vi "4Pi Focus Lock_ids_v1.vi"(7 "Calling VI Ref":refnum<vi>) -> ()   [LabVIEW 2021]
uses:
  4Pi Focus Lock Controls/4Pi Focus Lock - Notifier Type.ctl
  4Pi Focus Lock Controls/4Pi Focus Lock - Actions.ctl
  <vilib>/vision/Image Controls.llb/IMAQ Image.ctl
  <vilib>/Utility/miscctls.llb/LVPointTypeDef.ctl
  Hardware Configuration/Hardware Configuration Controls/Device Type.ctl
  Hardware Configuration/Hardware Configuration Controls/Device Function.ctl
  4Pi Objective Lock - EMBL/4Pi Objective Lock Type Defs/4Pi Obj Lock - Camera Settings.ctl
  Device Library/Cameras/Camera Controls/Generic Camera ROI.ctl
  Device Library/Cameras/Camera Controls/Generic Camera Actions.ctl
  Device Manager/Common Device Queue/Common Device Controls/Common Device Actions.ctl
  Device Library/Stages/Stages Controls/Stage Actions.ctl
  <vilib>/addons/control/pid/pid.llb/PID (DBL).vi
  <vilib>/vision/NI_Vision_Development_Module.lvlib
  <vilib>/addons/control/pid/NI_PID_pid.lvlib
panel:
  in  "Main Tab":enum32{"Acquisition", "Settings", "Gauss fit"}(tab)
  in  "Start Lock":bool
  out "Z Target and Fit Value (µm)":T1(graph)
  out "Stage Position (µm)":dbl=1.0 format="%.2g"
  out "Target Z (µm)":dbl=1.0 format="%.3g"
  out "Measured Z (µm)":dbl=1.0 format="%.3g"
  out "dt (s)":dbl format="%.3f"
  out "dz":dbl format="%.2f"
  out "Z Move":bool
  out "Measured X Position cc (px)":dbl=1.0 format="%.3g"
  out "Measured Y Position cc (px)":dbl=1.0 format="%.3g"
  out "Target Y Position cc (px)":dbl=1.0 format="%.3g"
  out "Target X Position cc (px)":dbl=1.0 format="%.3g"
  out "cc max":dbl=1.0 format="%.3g"
  out "X Y Fit Value (µm)":cluster{dbl, dbl, dbl, dbl, dbl}(graph)
  out "CC Max":cluster{" cc max":dbl}(graph)
  in  "Camera Settings":bool
  in  "Set Camera ROI":bool
  in  "P (Proportional)":dbl=2.0
  in  "I (Integral)":dbl
  in  "D (Derivative)":dbl
  in  "Z Correction Active":bool=TRUE
  in  "Z Move Limit (µm)":dbl=2.0
  in  "Z Drift Threshold (µm)":dbl=2.0
  in  "Sample Z Step Size (µm)":dbl=2.0
  in  "Sample Z Step No.":u32=2
  in  "Update Scale Factor":dbl=2.0
  in  "Frame Accumulation":u32=5
  in  "Pixe Size in XY (µm)":dbl=1.0
  out "Target sx/sy":dbl=1.0 format="%.3g"
  out "Target X Position G (px)":dbl=1.0 format="%.3g"
  out "Target Y Position G (px)":dbl=1.0 format="%.3g"
  out "Measured sx/sy":dbl=1.0 format="%.3g"
  out "Measured X Position G (px)":dbl=1.0 format="%.3g"
  out "Measured Y Position G (px)":dbl=1.0 format="%.3g"
  in  "Metric scale sx/sy":dbl=0.25
  in  "Quit":bool
  # "Z Drift Settings"
  # "PID Control Values"
  # "General Settings"
  # "Conversion to micron"
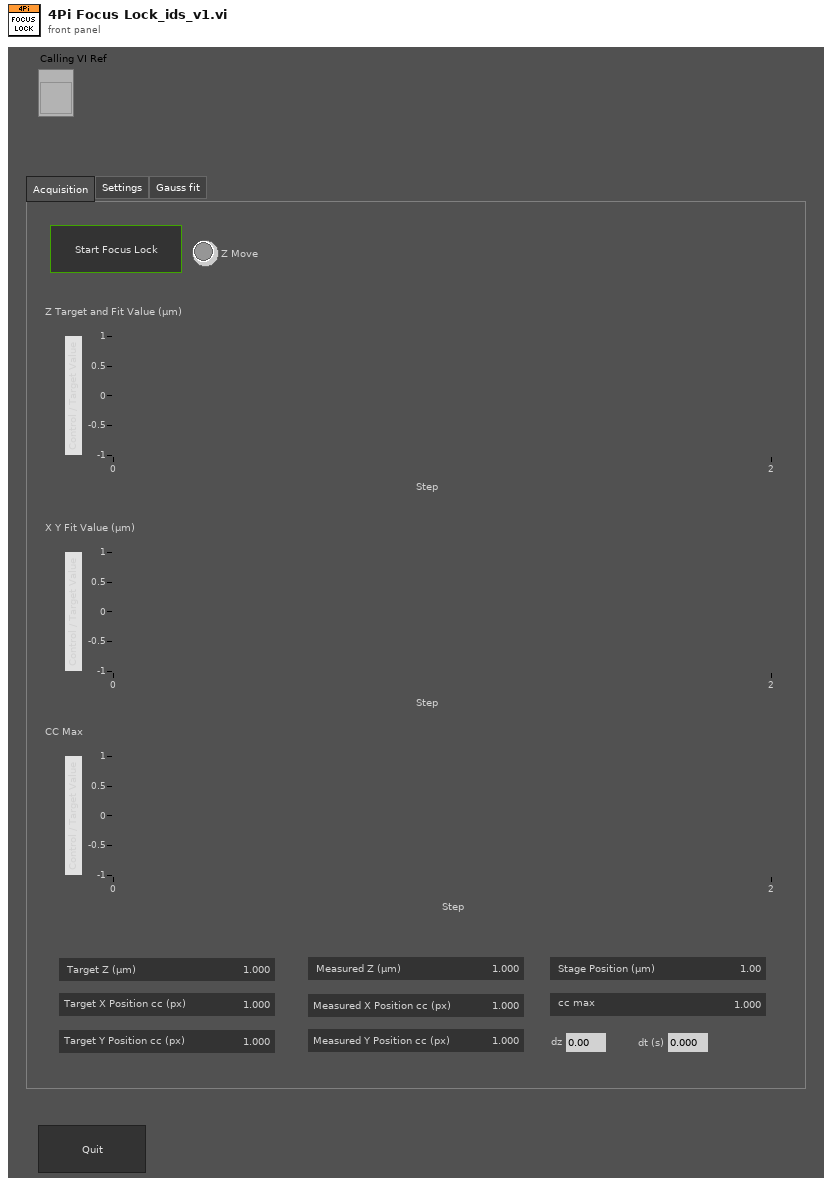
[diagram p1: front panel]
types:
  T1 = cluster{"Target 01":dbl, dbl, dbl, "Current 1":dbl, "Current 2":dbl, "Stage Position":dbl}
  T2 = typedef "4Pi Obj Lock - Camera Settings.ctl" = cluster{"Exposure Time (s)":dbl, "H Offset":u16, "V Offset":u16, "H Width":u16, "V Width":u16}
  T3 = typedef "Device Function.ctl" = enum16{"Primary", "Secondary", "Overview", "Wide Field Drift Correction", "642 nm Excitation", "560 nm Excitation", "940 nm Excitation", "546 nm Excitation", "488 nm Excitation", "405 nm Excitation", "Objective Drift Correction", "4Pi Focus Lock", "4Pi Objective Lock", "Objective XY", "Objective Z", "Sample XY", "Sample Coarse Z", "Sample Z", "4Pi Lower", "4Pi Upper", "Em Small", "Em Large", "Ex Small", "Ex Large", "Mojo", "Adj Cavity", "Line Scanning", "Alert"}
  T4 = typedef "Device Type.ctl" = enum16{"AOTF", "Camera", "Deformable Mirror", "Laser", "Flip Mirror", "Shutter", "Stage", "Waveform", "FPGA", "Email"}
  T5 = enum16{"Always On", "Always Off", "Off While Running"}
  T6 = typedef "LVPointTypeDef.ctl" = cluster{"Horizontal":i16, "Vertical":i16}
  T7 = typedef "4Pi Focus Lock - Actions.ctl" = enum16{"Idle", "Start Lock", "Restart Lock", "Get Target Position", "Get Ref Stack", "Cal Ref FFT", "Get Target Position Gauss", "Move To Init Z", "Start Primary Camera", "Get Current Position Gauss", "Get Current Position", "Get Current XY Position", "Get Current Position 1", "Get Actual Position", "Check Drift Gauss", "Check Drift", "Move Z", "Update Plots", "Delay", "Abort", "Exit Loop", "Quit"}
  T8 = typedef "4Pi Focus Lock - Notifier Type.ctl" = cluster{"Actions":T7, "Z Drift Threshold":dbl, "Z Stage Move Limit (µm)":dbl, "Abort If Error":bool, "Z Correction Active":bool, "PID Values":dbl[], "Running?":bool, "Update Delay (ms)":i32, "Z Step Size (µm)":dbl, "Z Step No.":u32, "No. of Frames":u32, "Ref Stack (SGL)":T9[], "Cur Image (SGL)":T9, "CC Image (SGL) ":T9, "Sample Z (µm)":dbl[], "Initial Z Position (µm)":dbl, "Ref FFT Stack (CSG)":T9[], "Tmp Image FFT (CSG) ":T9[], "CC Image Max (SGL)":T9}
  T9 = typedef "IMAQ Image.ctl" = refnum<image>
  T10 = typedef "Image Type" = u32
  T11 = typedef "Generic Camera Actions.ctl" = enum16{"Status", "Live Preview", "Capture", "Abort", "Set Exposure Time (s)", "Get Exposure Time (s)", "Record Settings", "Set ROI", "Get ROI", "Defect Correction On/Off", "Cooler On/Off", "Fan On/Off", "Quit"}
  T12 = typedef "Generic Camera ROI.ctl" = cluster{"H_Offset":u16, "V_Offset":u16, "H_Width":u16, "V_Width":u16}
  T13 = typedef "Common Device Actions.ctl" = enum16{"Specific Action", "Open Front Panel", "Close Front Panel", "Quit", "Quit All"}
  T14 = cluster{"Target 01":dbl, dbl, dbl, "Current 1":dbl, "Current 2":dbl, "Stage Position":dbl}[]
  T15 = typedef "Stage Actions.ctl" = enum16{"Get Position", "SERVO OFF", "SERVO ON", "SERVO ON/OFF", "MVR", "MOVE", "HALT", "ONTARGET", "ERROR", "REFERENCE", "INIT", "VELOCITY", "STATUS", "EXIT", "HOME", "ZEROPOS", "NANOPOS", "ANALOG", "QUIT"}
  T16 = typedef "Stage Status.ctl" = enum16{"Error", "Abort", "Busy", "On Target"}
  T17 = typedef "2D Gaussian - Best Fit Parameters.ctl" = cluster{"Amplitude":dbl, "X Position":dbl, "Y Position":dbl, "X Width":dbl, "Y Width":dbl, "Offset":dbl}
  T18 = cluster{"PID Values[0]":dbl, "PID Values[1]":dbl, "PID Values[2]":dbl}
  T19 = typedef "LVRectTypeDef.ctl" = cluster{"Left":i16, "Top":i16, "Right":i16, "Bottom":i16}
  T20 = typedef "LVBoundsTypeDef.ctl" = cluster{"Width":u32, "Height":u32}
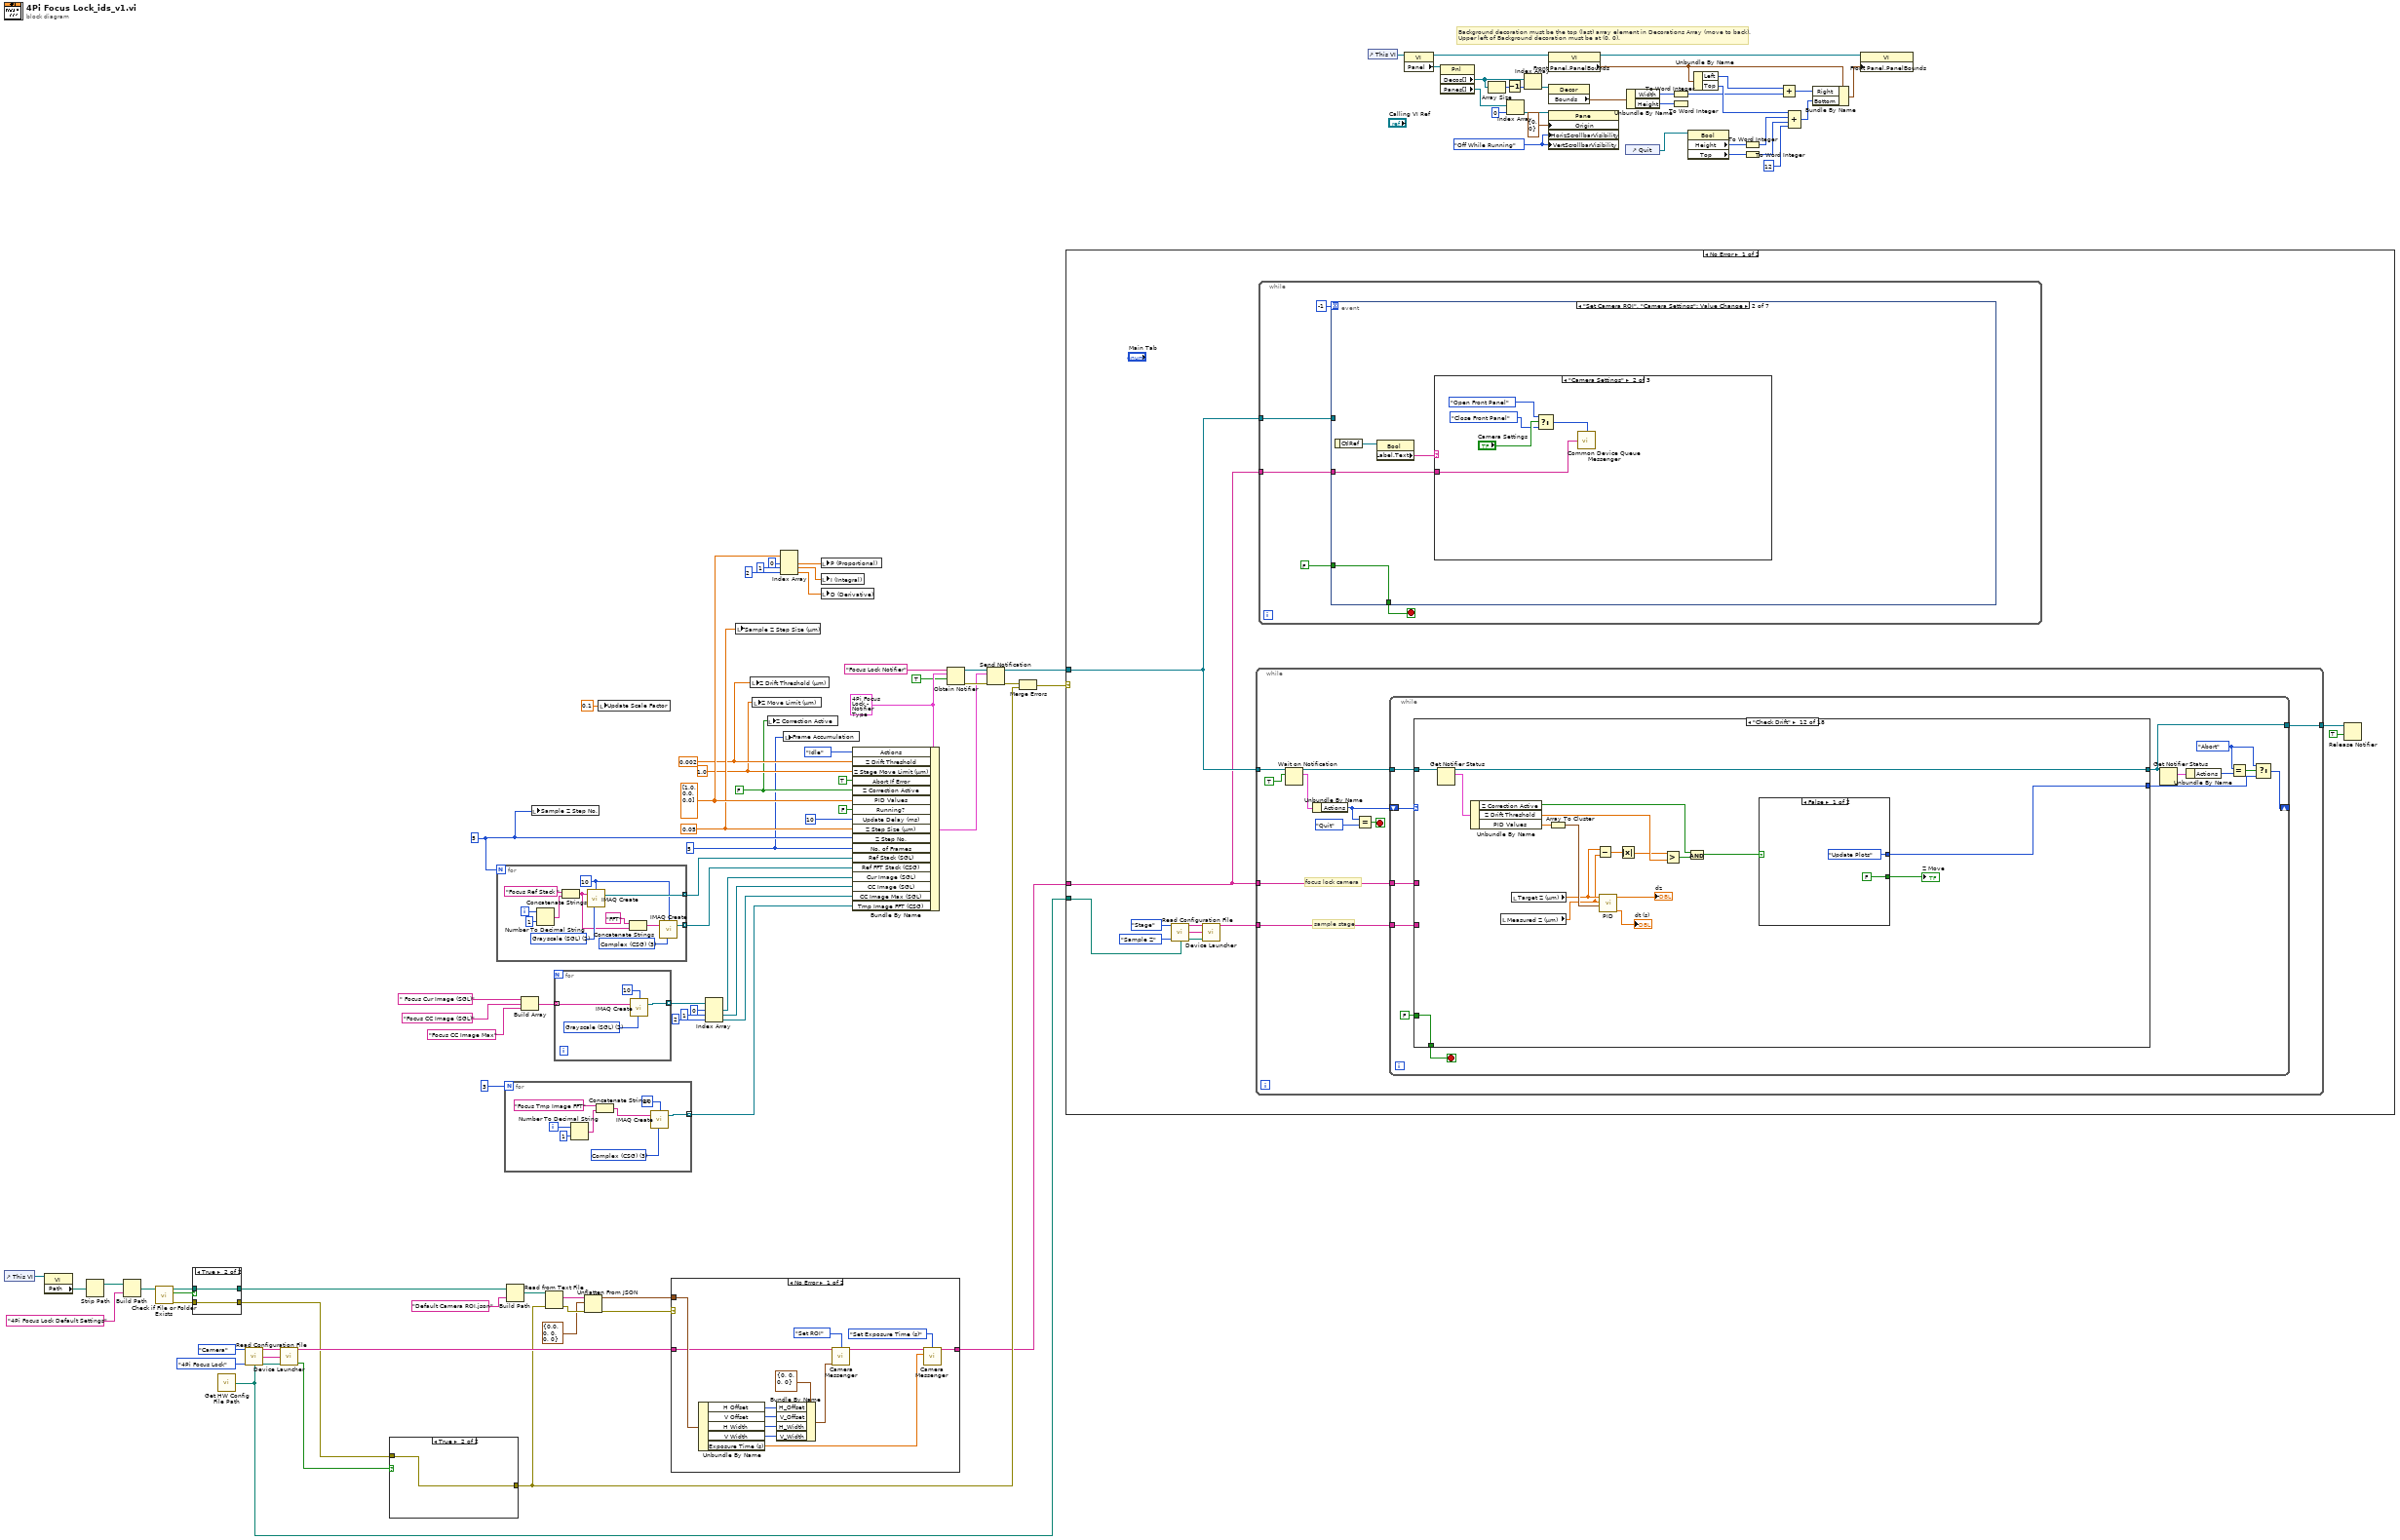
[diagram p0: block diagram]
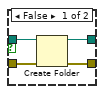
[diagram p2: hidden frame]
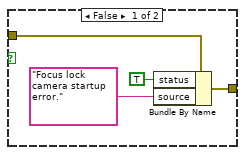
[diagram p3: hidden frame]
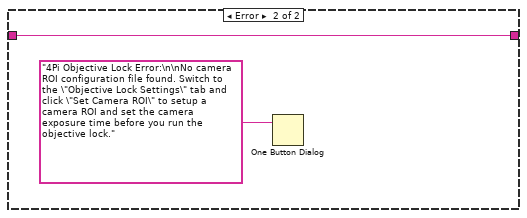
[diagram p4: hidden frame]
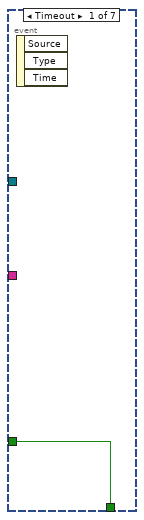
[diagram p5: hidden frame]
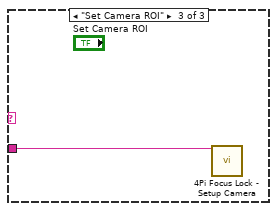
[diagram p7: hidden frame]
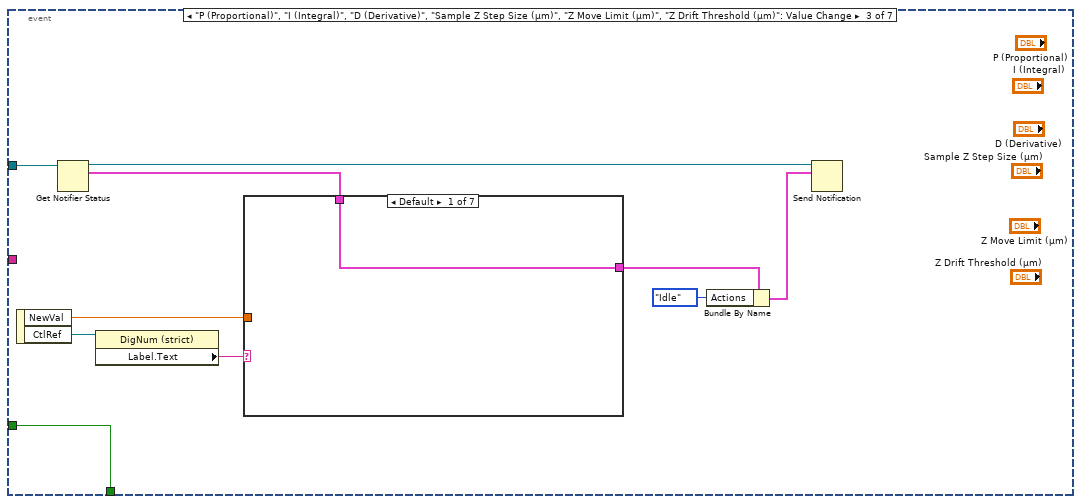
[diagram p8: hidden frame]
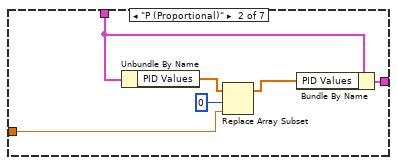
[diagram p9: hidden frame]
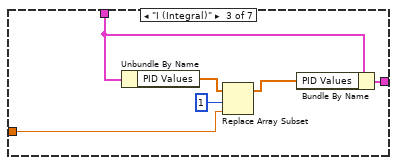
[diagram p10: hidden frame]
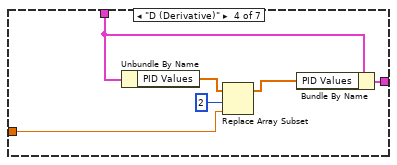
[diagram p11: hidden frame]
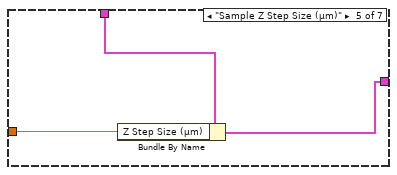
[diagram p12: hidden frame]
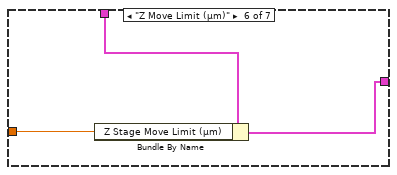
[diagram p13: hidden frame]
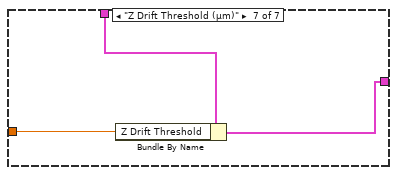
[diagram p14: hidden frame]
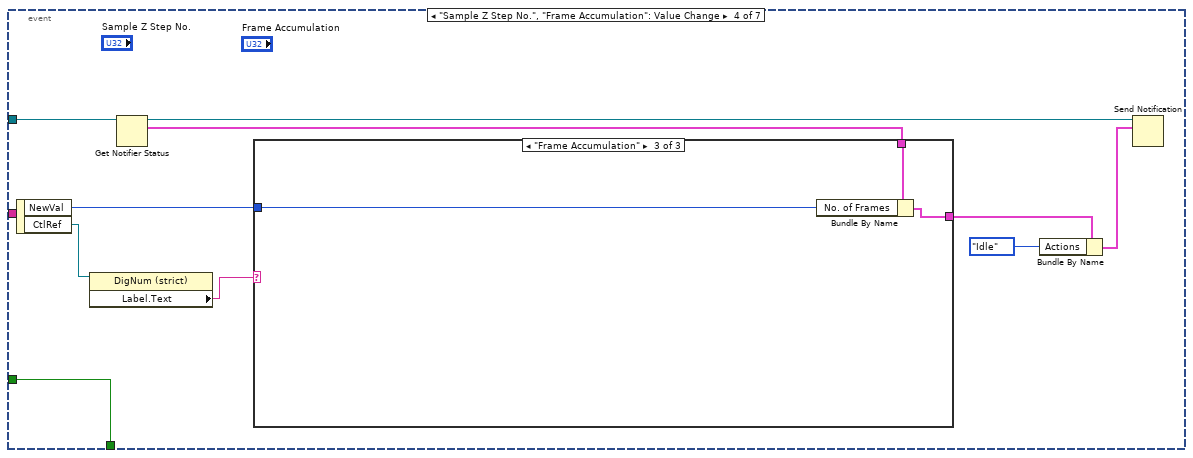
[diagram p15: hidden frame]
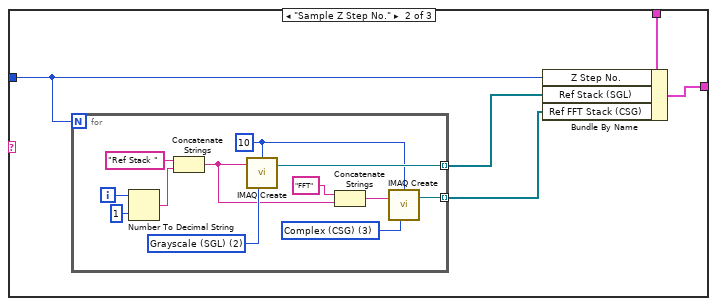
[diagram p17: hidden frame]
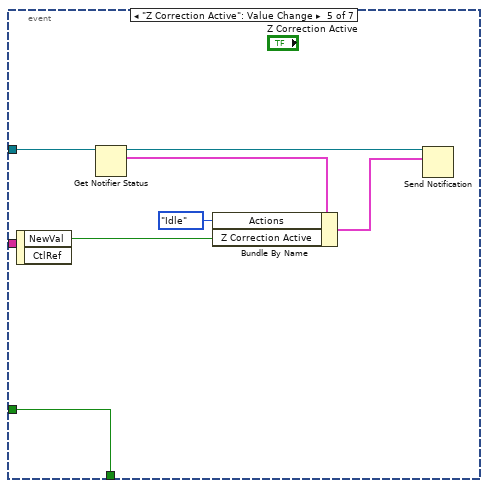
[diagram p18: hidden frame]
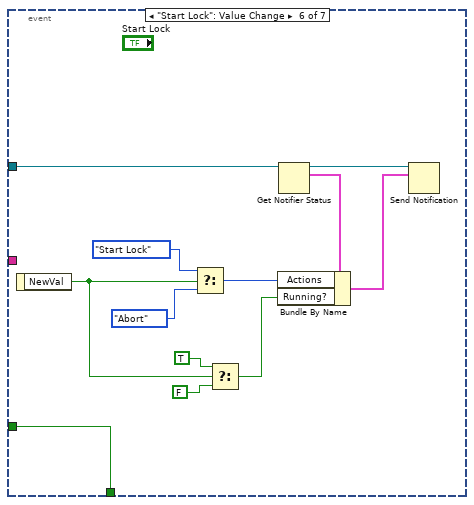
[diagram p19: hidden frame]
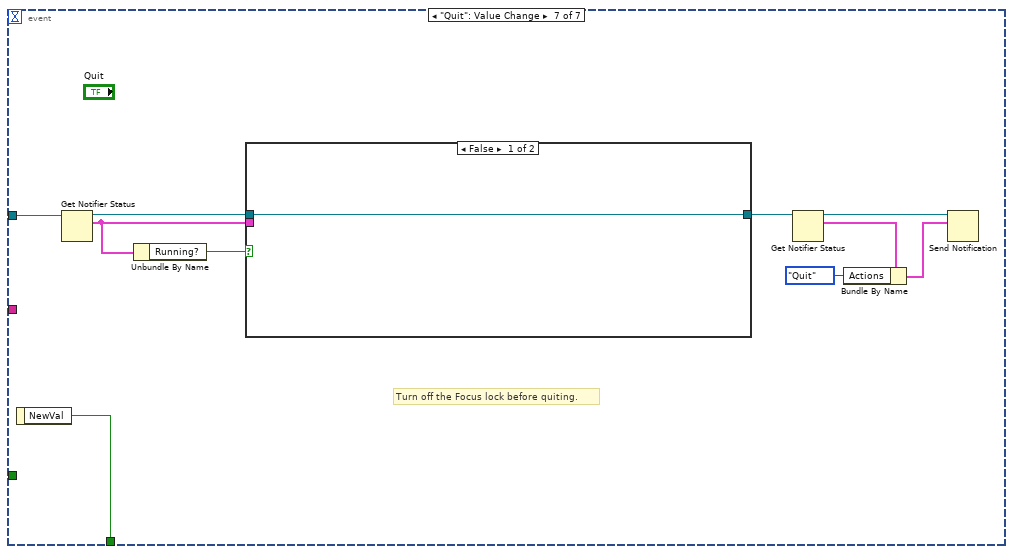
[diagram p20: hidden frame]
diagram:
  w39 = T5."Off While Running" ("Vertical Scrollbar Visibility")
  w57 = u32 5 ("No. of Frames")
  w80 = u32 5 ("Z Step No.")
  w84 = 0.05 ("Z Step Size (µm)")
  w88 = dbl[] [1.0, 0.0, 0.0] ("PID Values")
  w61 = FALSE ("Z Correction Active")
  w67 = 1.0 ("Z Stage Move Limit (µm)")
  w68 = 0.002 ("Z Drift Threshold")
  w70 = T8 {"Actions"=enum."Idle", "Z Drift Threshold"=0.05, "Z Stage Move Limit (µm)"=1.0, "Abort If Error"=FALSE, "Z Correction Active"=FALSE, "PID Values"=[], "Running?"=FALSE, "Update Delay (ms)"=0, "Z Step Size (µm)"=2.0, "Z Step No."=2, "No. of Frames"=0, "Ref Stack (SGL)"=[], "Cur Image (SGL)"=refnum, "CC Image (SGL) "=refnum, "Sample Z (µm)"=[], "Initial Z Position (µm)"=0.0, "Ref FFT Stack (CSG)"=[], "Tmp Image FFT (CSG) "=[], "CC Image Max (SGL)"=refnum} ("4Pi Focus Lock")
  # "Background decoration must be the top (last) array element in Decorations Array (move to back).\nUpper left of Background decoration must be at (0, 0)."
  n1 = control-ref of="This VI"() -> (w13:refnum<vi>)
  n2 = property class="VI"(reference=w13) -> ("Path"=w11:path)  [unwired: 1 in, 2 out]
  n3 = Strip Path(path=w11) -> (stripped path=w10:path)  [unwired: 1 out]
  n4 = Build Path(base path=w10, name or relative path="4Pi Focus Lock Default Settings") -> (appended path=w9:path)
  n5 = call <vilib>:"Check if File or Folder Exists.vi"("path"=w9) -> ("error out"=w6:errorcluster, "file or folder exists?"=w8:bool, "dup path"=w7:path)  [unwired: 8 in]
  n6 = case shown="True" w8 {
    tunnel: w7 -> [w102 w104]
    tunnel: [w101 w104] -> w4
    tunnel: w6 -> [w100 w103]
    tunnel: [w99 w103] -> w5
    frame False {
      n7 = Create Folder(path (use dialog)=w102, error in=w100) -> (created path=w101:path, error out=w99:errorcluster)  [unwired: 1 in, 1 out]
    }
    frame True {
    }
  }
  n8 = call "Get HW Config File Path.vi"() -> ("File Path"=w2:path)  [unwired: 14 in, 1 out]
  n9 = call "Read Configuration File.vi"("Device Type"=Device_Type."Camera", "Device Function"=Device_Function."4Pi Focus Lock", "Config File Path"=w2) -> ("Unique Notifier Name"=w23:string, "Device Ports/IDs/Channels"=w25:string[], "Device Engine Path"=w24:path)  [unwired: 9 in, 1 out]
  n10 = call "Device Launcher.vi"("Notifier Name"=w23, "Device Ports/IDs/Channels"=w25, "Device Engine Path"=w24) -> ("Notifier Name"=w17:string, "Running?"=w20:bool)  [unwired: 11 in]
  n11 = case shown="True" w20 {
    tunnel: w5 -> [w108 w109]
    tunnel: [w105 w109] -> w3
    frame False {
      n12 = Bundle By Name(cluster=w108, "status"=TRUE, "source"="Focus lock camera startup error." ("name or relative path")) -> (w105:errorcluster)
    }
    frame True {
    }
  }
  n13 = for {
    N: w80 -> [_]
    tunnel: [w121] -> w79 mode=indexing
    tunnel: [w110] -> w64 mode=indexing
    i -> [w120]
    w115 = T10 3 items=["Grayscale (U8)", "Grayscale (I16)", "Grayscale (SGL)", "Complex (CSG)", "RGB (U32)", "HSL (U32)", "RGB (U64)", "Grayscale (U16)"] ("Image Type")
    w116 = T10 2 items=["Grayscale (U8)", "Grayscale (I16)", "Grayscale (SGL)", "Complex (CSG)", "RGB (U32)", "HSL (U32)", "RGB (U64)", "Grayscale (U16)"] ("Image Type")
    w112 = 10 ("Border Size")
    n14 = Number To Decimal String(number=w120, width (-)=i16 1) -> (decimal integer string=w118:string)
    n15 = Concatenate Strings("Focus Ref Stack " ("string"), w118) -> (w111:string)
    n16 = call "IMAQ Create"("Border Size"=w112, "Image Name"=w111, "Image Type"=w116) -> ("New Image"=w121:T9)  [unwired: 2 in, 1 out]
    n17 = Concatenate Strings("FFT" ("string"), w111) -> (w114:string)
    n18 = call "IMAQ Create"("Border Size"=w112, "Image Name"=w114, "Image Type"=w115) -> ("New Image"=w110:T9)  [unwired: 2 in, 1 out]
  }
  n19 = for {
    N: 3 -> [_]
    tunnel: [w127] -> w62 mode=indexing
    i -> [w123]
    w128 = T10 3 items=["Grayscale (U8)", "Grayscale (I16)", "Grayscale (SGL)", "Complex (CSG)", "RGB (U32)", "HSL (U32)", "RGB (U64)", "Grayscale (U16)"] ("Image Type")
    n20 = Number To Decimal String(number=w123, width (-)=i16 1) -> (decimal integer string=w126:string)
    n21 = Concatenate Strings("Focus Tmp Image FFT" ("Image Name"), w126) -> (w122:string)
    n22 = call "IMAQ Create"("Border Size"=10, "Image Name"=w122, "Image Type"=w128) -> ("New Image"=w127:T9)  [unwired: 2 in, 1 out]
  }
  n23 = Build Path(base path=w4, name or relative path="Default Camera ROI.json") -> (appended path=w15:path)
  n24 = Build Array(" Focus Cur Image (SGL)" ("Image Name"), "Focus CC Image (SGL)" ("Image Name"), "Focus CC Image Max" ("element")) -> (w74:string[])
  n25 = local write "Sample Z Step No."(w80) -> ()
  n26 = Read from Text File(file (use dialog)=w15, error in=w3) -> (text=w27:string, error out=w26:errorcluster)  [unwired: 2 in, 2 out]
  n27 = for {
    tunnel: w74 -> [w131] mode=indexing
    tunnel: [w130] -> w73 mode=indexing
    w132 = T10 2 items=["Grayscale (U8)", "Grayscale (I16)", "Grayscale (SGL)", "Complex (CSG)", "RGB (U32)", "HSL (U32)", "RGB (U64)", "Grayscale (U16)"] ("Image Type")
    n28 = call "IMAQ Create"("Border Size"=10, "Image Name"=w131, "Image Type"=w132) -> ("New Image"=w130:T9)  [unwired: 2 in, 1 out]
  }
  n29 = Unflatten From JSON(JSON string=w27, type and defaults=T2 {"Exposure Time (s)"=0.0, "H Offset"=0, "V Offset"=0, "H Width"=0, "V Width"=0} ("Camera Settings"), error in (no error)=w26) -> (value=w16:T2, error out=w19:errorcluster)  [unwired: 4 in]
  n30 = local write "Update Scale Factor"(0.1 ("Update Scale Factor")) -> ()
  n31 = case shown="No Error" w19 {
    tunnel: w17 -> [w137 w148]
    tunnel: w16 -> [w146 _]
    tunnel: [w134 w148] -> w1
    frame No Error {
      n32 = Unbundle By Name(w146) -> ("H Offset"=w141:u16, "V Offset"=w142:u16, "H Width"=w143:u16, "V Width"=w144:u16, "Exposure Time (s)"=w136:dbl)
      n33 = Bundle By Name(cluster=T12 {"H_Offset"=0, "V_Offset"=0, "H_Width"=0, "V_Width"=0} ("General Camera ROI"), "H_Offset"=w141, "V_Offset"=w142, "H_Width"=w143, "V_Width"=w144) -> (w140:T12)
      n34 = call "Camera Messenger.vi"("Notifier Name"=w137, "General Camera Actions"=Generic_Camera_Actions."Set ROI", "Camera ROI"=w140) -> ("Notifier Name Dup"=w135:string)  [unwired: 7 in, 5 out]
      n35 = call "Camera Messenger.vi"("Notifier Name"=w135, "General Camera Actions"=Generic_Camera_Actions."Set Exposure Time (s)", "Exposure Time (s)"=w136) -> ("Notifier Name Dup"=w134:string)  [unwired: 7 in, 5 out]
    }
    frame Error {
      n36 = One Button Dialog(message="4Pi Objective Lock Error:\n\nNo camera ROI configuration file found. Switch to the \"Objective Lock Settings\" tab and click \"Set Camera ROI\" to setup a camera ROI and set the camera exposure time before you run the objective lock.") -> ()  [unwired: 1 in, 1 out]
    }
  }
  n37 = Index Array(array=w73, index #1=0 ("index"), index #2=1 ("index"), index #3=2 ("index")) -> (element #1=w72:T9, element #2=w71:T9, element #3=w58:T9)
  n38 = local write "Sample Z Step Size (µm)"(w84) -> ()
  n39 = local write "Z Drift Threshold (µm)"(w68) -> ()
  n40 = local write "Z Move Limit (µm)"(w67) -> ()
  n41 = local write "Z Correction Active"(w61) -> ()
  n42 = Index Array(array=w88, index #1=0 ("index"), index #2=1 ("index"), index #3=2 ("index")) -> (element #1=w87:dbl, element #2=w86:dbl, element #3=w85:dbl)
  n43 = local write "Frame Accumulation"(w57) -> ()
  n44 = local write "P (Proportional)"(w87) -> ()
  n45 = local write "I (Integral)"(w86) -> ()
  n46 = local write "D (Derivative)"(w85) -> ()
  n47 = Bundle By Name(cluster=w70, "Actions"=4Pi_Focus_Lock_-_Actions."Idle", "Z Drift Threshold"=w68, "Z Stage Move Limit (µm)"=w67, "Abort If Error"=TRUE, "Z Correction Active"=w61, "PID Values"=w88, "Running?"=FALSE, "Update Delay (ms)"=10, "Z Step Size (µm)"=w84, "Z Step No."=w80, "No. of Frames"=w57, "Ref Stack (SGL)"=w79, "Ref FFT Stack (CSG)"=w64, "Cur Image (SGL)"=w72, "CC Image (SGL)"=w71, "CC Image Max (SGL)"=w58, "Tmp Image FFT (CSG)"=w62) -> (w65:T8)
  n48 = Obtain Notifier(name (unnamed)="Focus Lock Notifier", notification data type=w70, create if not found? (T)=TRUE) -> (notifier out=w93:refnum<notifier>, error out=w92:errorcluster)  [unwired: 1 in, 1 out]
  n49 = Send Notification(notification=w65, notifier=w93, error in (no error)=w92) -> (notifier out=w81:refnum<notifier>, error out=w83:errorcluster)
  n50 = Merge Errors(w83, w3) -> (w82:errorcluster)
  n51 = case shown="No Error" w82 {
    tunnel: w2 -> [w150 _]
    tunnel: w81 -> [w153 _]
    tunnel: w1 -> [w149 _]
    frame No Error {
      n52 = call "Read Configuration File.vi"("Device Type"=Device_Type."Stage", "Device Function"=Device_Function."Sample Z", "Config File Path"=w150) -> ("Unique Notifier Name"=w159:string, "Device Ports/IDs/Channels"=w157:string[], "Device Engine Path"=w156:path)  [unwired: 9 in, 1 out]
      n53 = call "Device Launcher.vi"("Notifier Name"=w159, "Device Ports/IDs/Channels"=w157, "Device Engine Path"=w156) -> ("Notifier Name"=w154:string)  [unwired: 11 in, 1 out]
      n54 = while {
        tunnel: w153 -> [w300]
        tunnel: w149 -> [w294]
        tunnel: w154 -> [w293]
        tunnel: [w291] -> w151
        stop <- w296 stop-if-true
        # "sample stage"
        # "focus lock camera"
        n55 = Wait on Notification(notifier=w300, ignore previous (F)=TRUE) -> (notifier out=w292:refnum<notifier>, notification=w298:T8)  [unwired: 2 in, 2 out]
        n56 = Unbundle By Name(w298) -> ("Actions"=w295:T7)
        n57 = Equal?(x=w295, y=4Pi_Focus_Lock_-_Actions."Quit") -> (x = y?=w296:bool)
        n58 = while {
          tunnel: w294 -> [w312]
          tunnel: w293 -> [w311]
          tunnel: w292 -> [w310]
          shift-right: [w304] -> _
          shift-left: w295 -> [w313]
          tunnel: [w301] -> w291
          stop <- w303 stop-if-true
          w306 = 4Pi_Focus_Lock_-_Actions."Abort" ("y")
          n59 = case shown="\"Check Drift\"" w313 {
            tunnel: w312 -> [_ w336 _ w422 _ _ w498 w538 _ w592 w624 _ _ _ _ w777 _ _]
            tunnel: w311 -> [_ w343 w400 w415 _ w467 _ _ _ _ _ _ _ w707 w737 _ _ _]
            tunnel: w310 -> [w314 w352 w401 w423 w460 w472 w499 w551 w570 w619 w639 w668 w692 w712 w771 w778 w785 w788]
            tunnel: [4Pi_Focus_Lock_-_Actions."Exit Loop" ("y") w330 4Pi_Focus_Lock_-_Actions."Get Ref Stack" ("y") w416 4Pi_Focus_Lock_-_Actions."Move To Init Z" ("y") 4Pi_Focus_Lock_-_Actions."Get Target Position Gauss" ("y") w495 w541 4Pi_Focus_Lock_-_Actions."Get Current Position Gauss" ("y") w593 4Pi_Focus_Lock_-_Actions."Check Drift" ("y") w651 w680 w697 4Pi_Focus_Lock_-_Actions."Get Current Position" ("y") 4Pi_Focus_Lock_-_Actions."Exit Loop" ("y") 4Pi_Focus_Lock_-_Actions."Exit Loop" ("y") 4Pi_Focus_Lock_-_Actions."Quit" ("y")] -> w305
            tunnel: [w314 w338 w388 w418 w457 w470 w488 w548 w566 w618 w634 w661 w688 w705 w760 w774 w785 w788] -> w301
            tunnel: [w315 w337 w387 w417 w455 w468 w489 w547 w564 w614 w633 w660 w687 w704 w759 w773 TRUE TRUE] -> w303
            tunnel: FALSE -> [w315 w337 w387 w417 w455 w468 w489 w547 w564 w614 w633 w660 w687 w704 w759 w773 _ _]
            frame "Idle", Default {
            }
            frame "Start Lock" {
              n60 = Get Notifier Status(notifier=w352) -> (notifier out=w339:refnum<notifier>, current notification=w342:T8)  [unwired: 1 in, 3 out]
              n61 = Unbundle By Name(w342) -> ("Z Step No."=w349:u32, "Ref Stack (SGL)"=w348:T9[])
              n62 = Unbundle By Name(w342) -> ("Cur Image (SGL)"=w347:T9)
              n63 = call "Stages Messenger.vi"("Stage Notifier Name"=w343, "Actions"=Stage_Actions."Get Position") -> ("Positions"=w344:dbl[])  [unwired: 9 in, 4 out]
              n64 = Index Array(array=w344, index=0) -> (element=w341:dbl)
              n65 = call "Camera Messenger.vi"("Notifier Name"=w336, "General Camera Actions"=Generic_Camera_Actions."Get ROI", "Camera ROI"=T12 {"H_Offset"=0, "V_Offset"=0, "H_Width"=0, "V_Width"=0} ("General Camera ROI")) -> ("Notifier Name Dup"=w335:string, "Camera ROI"=w357:T12)  [unwired: 7 in, 4 out]
              n66 = Unbundle By Name(w357) -> ("H_Width"=w356:u16, "V_Width"=w354:u16)
              n67 = To Long Integer(number=w356) -> (32bit integer=w355:i32)
              n68 = To Long Integer(number=w354) -> (32bit integer=w353:i32)
              n69 = Initialize Array(sgl 0.0 ("element"), w355, w353) -> (w320:sgl[][])
              n70 = for {
                N: w349 -> [_]
                tunnel: w320 -> [w368]
                tunnel: w348 -> [w369] mode=indexing
                n71 = call "IMAQ ArrayToImage"("Image Pixels (Float)"=w368, "Image"=w369) -> ()  [unwired: 8 in, 2 out]
              }
              n72 = call "IMAQ ArrayToImage"("Image Pixels (Float)"=w320, "Image"=w347) -> ()  [unwired: 8 in, 2 out]
              n73 = call "Camera Messenger.vi"("Notifier Name"=w335, "General Camera Actions"=Generic_Camera_Actions."Live Preview") -> ("Notifier Name Dup"=w334:string)  [unwired: 8 in, 5 out]
              n74 = while {
                tunnel: w334 -> [w366]
                tunnel: [w361] -> w333
                i -> [w365]
                stop <- w362 stop-if-true
                n75 = call "Camera Messenger.vi"("Notifier Name"=w366, "General Camera Actions"=Generic_Camera_Actions."Status") -> ("Running?"=w363:bool)  [unwired: 8 in, 5 out]
                n76 = Greater?(x=w365, y=3000) -> (0:w361:bool)
                n77 = Or(x=w363, y=w361) -> (x .or. y?=w362:bool)
                n78 = Wait (ms)(milliseconds to wait=u32 1) -> ()  [unwired: 1 out]
              }
              n79 = Array Size(array=w320) -> (size(s)=w326:i32[])
              n80 = Bundle By Name(cluster=w342, "Initial Z Position (µm)"=w341) -> (w340:T8)
              n81 = To Double Precision Float(number=w326) -> (double precision float=w329:dbl[])
              n82 = Divide(x=w329, y=2.0 ("index")) -> (x/y=w327:dbl[])
              n83 = Round Toward -Infinity(1:w327) -> (0:w325:dbl[])
              n84 = Send Notification(notification=w340, notifier=w339) -> (notifier out=w338:refnum<notifier>)  [unwired: 1 in, 1 out]
              n85 = Index Array(array=w325, index #1=0 ("index"), index #2=1 ("index")) -> (element #1=→"Target Y Position cc (px)":dbl, element #2=→"Target X Position cc (px)":dbl)
              n86 = property on="Z Target and Fit Value (µm)" class="WFChart (strict)"("History Data"=T14 []) -> ()  [unwired: 2 in, 2 out]
              n87 = Select(t=4Pi_Focus_Lock_-_Actions."Exit Loop" ("y"), s=w333, f=4Pi_Focus_Lock_-_Actions."Get Target Position") -> (s? t:f=w330:T7)
              n88 = property on="CC Max" class="WFChart (strict)"("History Data"=cluster{" cc max":dbl}[] []) -> ()  [unwired: 2 in, 2 out]
              n89 = property on="X Y Fit Value (µm)" class="WFChart (strict)"("History Data"=cluster{dbl, dbl, dbl, dbl, dbl}[] []) -> ()  [unwired: 2 in, 2 out]
            }
            frame "Get Target Position" {
              w394 = 0.0 ("Target Z (µm)")
              n90 = Get Notifier Status(notifier=w401) -> (notifier out=w392:refnum<notifier>, current notification=w397:T8)  [unwired: 1 in, 3 out]
              n91 = Unbundle By Name(w397) -> ("Z Step No."=w386:u32, "Z Step Size (µm)"=w385:dbl, "Z Stage Move Limit (µm)"=w383:dbl)
              n92 = Unbundle By Name(w397) -> ("Z Step No."=w378:u32, "Z Step Size (µm)"=w395:dbl)
              n93 = Divide(x=w386, y=2.0) -> (x/y=w376:dbl)
              n94 = Round Toward -Infinity(1:w376) -> (0:w375:dbl)
              n95 = Multiply(x=w375, y=w385) -> (x*y=w380:dbl)
              n96 = Decrement(x=w378) -> (x-1=w377:u32)
              n97 = Negate(x=w380) -> (-x=w379:dbl)
              n98 = Negate(x=w383) -> (-x=w384:dbl)
              n99 = In Range and Coerce(upper limit=w383, x=w379, lower limit=w384) -> (coerced(x)=w381:dbl)  [unwired: 1 out]
              n100 = Add(x=w394, y=w381) -> (x+y=w382:dbl)
              n101 = Build Array(w382) -> (w396:dbl[])
              n102 = for {
                N: w377 -> [_]
                tunnel: w395 -> [w410]
                shift-right: [w411] -> w393
                shift-left: w396 -> [w412]
                shift-right: [w408] -> _
                shift-left: w382 -> [w409]
                n103 = Add(x=w409, y=w410) -> (x+y=w408:dbl)
                n104 = Build Array (concatenate)(w412, w408) -> (w411:dbl[])
              }
              n105 = Build Array(w381) -> (w398:dbl[])
              n106 = call "Stages Messenger.vi"("Stage Notifier Name"=w400, "Actions"=Stage_Actions."MVR", "Setpoint"=w398, "Axis"=bool[] [TRUE], "Exit While Busy?"=FALSE) -> ("Stage Notifier Name (Dup)"=w373:string, "Status"=w374:T16)  [unwired: 6 in, 3 out]
              n107 = case shown="Default" w374 {
                tunnel: [w406] -> w372
                tunnel: w373 -> [w406]
                frame Default {
                  n108 = Wait (ms)(milliseconds to wait=u32 350) -> ()  [unwired: 1 out]
                }
              }
              n109 = Bundle By Name(cluster=w397, "Sample Z (µm)"=w393) -> (w391:T8)
              n110 = call "Stages Messenger.vi"("Stage Notifier Name"=w372, "Actions"=Stage_Actions."Get Position") -> ("Positions"=w370:dbl[])  [unwired: 9 in, 4 out]
              n111 = Index Array(array=w370, index=0) -> (element=→"Stage Position (µm)":dbl)
              n112 = Send Notification(notification=w391, notifier=w392) -> (notifier out=w388:refnum<notifier>)  [unwired: 1 in, 1 out]
              "Target Z (µm)" <- w394
            }
            frame "Get Ref Stack" {
              n113 = Get Notifier Status(notifier=w423) -> (notifier out=w418:refnum<notifier>, current notification=w414:T8)  [unwired: 1 in, 3 out]
              n114 = Unbundle By Name(w414) -> ("Z Step No."=w421:u32, "Ref Stack (SGL)"=w420:T9[])
              n115 = Unbundle By Name(w414) -> ("No. of Frames"=w413:u32)
              n116 = Unbundle By Name(w414) -> ("Z Step Size (µm)"=w419:dbl)
              n117 = while {
                tunnel: w422 -> [w441]
                tunnel: w421 -> [w438]
                tunnel: w418 -> [w440]
                tunnel: [w428] -> w416
                tunnel: w420 -> [w427] mode=indexing
                tunnel: w419 -> [w426]
                tunnel: w415 -> [w425]
                tunnel: w413 -> [w424]
                i -> [w437]
                stop <- w433 stop-if-true
                n118 = flat-sequence {
                  tunnel: w441 -> [w445]
                  tunnel: w427 -> [w444]
                  tunnel: w424 -> [w443]
                  tunnel: w426 -> [w449]
                  tunnel: w425 -> [w448]
                  frame #0 {
                    n119 = To Unsigned Word Integer(number=w443) -> (unsigned 16bit integer=w442:u16)
                    n120 = call "Generic Camera Get New Camera Image.vi"("Camera Notifier Name"=w445, "Frames"=w442) -> ("Image - U16"=w447:u16[][])  [unwired: 11 in, 2 out]
                    n121 = To Single Precision Float(number=w447) -> (single precision float=w446:sgl[][])
                    n122 = call "IMAQ ArrayToImage"("Image Pixels (Float)"=w446, "Image"=w444) -> ()  [unwired: 8 in, 2 out]
                  }
                  frame #1 {
                    n123 = Build Array(w449) -> (w453:dbl[])
                    n124 = call "Stages Messenger.vi"("Stage Notifier Name"=w448, "Actions"=Stage_Actions."MVR", "Setpoint"=w453, "Axis"=bool[] [TRUE], "Exit While Busy?"=FALSE) -> ()  [unwired: 6 in, 5 out]
                  }
                  frame #2 {
                    n125 = Wait (ms)(milliseconds to wait=u32 350) -> ()  [unwired: 1 out]
                  }
                }
                n126 = Get Notifier Status(notifier=w440) -> (current notification=w432:T8)  [unwired: 1 in, 4 out]
                n127 = To Unsigned Long Integer(number=w437) -> (unsigned 32bit integer=w436:u32)
                n128 = Increment(x=w436) -> (x+1=w439:u32)
                n129 = Unbundle By Name(w432) -> ("Running?"=w435:bool)
                n130 = Greater Or Equal?(x=w439, y=w438) -> (x >= y?=w434:bool)
                n131 = Not(x=w435) -> (.not. x?=w431:bool)
                n132 = Or(x=w431, y=w434) -> (x .or. y?=w433:bool)
                n133 = Select(t=4Pi_Focus_Lock_-_Actions."Abort", s=w431, f=4Pi_Focus_Lock_-_Actions."Cal Ref FFT" ("y")) -> (s? t:f=w428:T7)
              }
            }
            frame "Cal Ref FFT" {
              n134 = Get Notifier Status(notifier=w460) -> (notifier out=w457:refnum<notifier>, current notification=w461:T8)  [unwired: 1 in, 3 out]
              n135 = Unbundle By Name(w461) -> ("Ref Stack (SGL)"=w458:T9[], "Ref FFT Stack (CSG)"=w459:T9[])
              n136 = for {
                tunnel: w459 -> [w462] mode=indexing
                tunnel: w458 -> [w463] mode=indexing
                n137 = call "4Pi Focus Lock - Norm FFT.vi"("FFT Image Dst"=w462, "Image In"=w463) -> ()  [unwired: 8 in, 2 out]
              }
            }
            frame "Move To Init Z" {
              n138 = Get Notifier Status(notifier=w472) -> (notifier out=w470:refnum<notifier>, current notification=w471:T8)  [unwired: 1 in, 3 out]
              n139 = Unbundle By Name(w471) -> ("Initial Z Position (µm)"=w465:dbl)
              n140 = flat-sequence {
                tunnel: w467 -> [w480]
                tunnel: [w479] -> w466
                tunnel: w465 -> [w475]
                tunnel: [w473] -> w464
                tunnel: w466 -> [w483]
                tunnel: w464 -> [w482]
                frame #0 {
                  n141 = call "Stages Messenger.vi"("Stage Notifier Name"=w480, "Actions"=Stage_Actions."Get Position") -> ("Stage Notifier Name (Dup)"=w479:string, "Positions"=w477:dbl[])  [unwired: 9 in, 3 out]
                  n142 = Index Array(array=w477, index=0) -> (element=w476:dbl)
                  n143 = Subtract(x=w475, y=w476) -> (x-y=w474:dbl)
                  n144 = Build Array(w474) -> (w473:dbl[])
                }
                frame #1 {
                  n145 = call "Stages Messenger.vi"("Stage Notifier Name"=w483, "Actions"=Stage_Actions."MVR", "Setpoint"=w482, "Axis"=bool[] [TRUE], "Exit While Busy?"=FALSE) -> ()  [unwired: 6 in, 5 out]
                }
                frame #2 {
                  n146 = Wait (ms)(milliseconds to wait=u32 350) -> ()  [unwired: 1 out]
                }
              }
            }
            frame "Get Target Position Gauss" {
              n147 = Get Notifier Status(notifier=w499) -> (notifier out=w513:refnum<notifier>, current notification=w502:T8)  [unwired: 1 in, 3 out]
              n148 = Unbundle By Name(w502) -> ("No. of Frames"=w497:u32)
              n149 = Bundle By Name(cluster=w502, "Running?"=TRUE) -> (w511:T8)
              n150 = Send Notification(notification=w511, notifier=w513) -> (notifier out=w488:refnum<notifier>)  [unwired: 1 in, 1 out]
              n151 = To Unsigned Word Integer(number=w497) -> (unsigned 16bit integer=w496:u16)
              n152 = call "Generic Camera Get New Camera Image.vi"("Camera Notifier Name"=w498, "Frames"=w496) -> ("Image - U16"=w501:u16[][])  [unwired: 11 in, 2 out]
              n153 = call "2D Gaussian - Fit Image U16.vi"("Image In (U16)"=w501) -> ("Best Fit Params"=w517:T17, "Error Out"=w507:errorcluster)  [unwired: 13 in]
              n154 = Unbundle By Name(w507) -> ("status"=w500:bool)
              n155 = Cluster To Array(cluster=w517) -> (array=w516:dbl[])
              n156 = Array Subset(array=w516, index=1, length=4) -> (w510:dbl[])
              n157 = Index Array(array=w510, index #1=0 ("index"), index #2=1 ("index"), index #3=2 ("index"), index #4=3 ("index")) -> (element #1=→"Target X Position G (px)":dbl, element #2=→"Target Y Position G (px)":dbl, element #3=w504:dbl, element #4=w503:dbl)
              n158 = Divide(x=w504, y=w503) -> (x/y=→"Target sx/sy":dbl)
              n159 = Select(t=4Pi_Focus_Lock_-_Actions."Abort" ("y"), s=w500, f=4Pi_Focus_Lock_-_Actions."Get Current Position") -> (s? t:f=w495:T7)
            }
            frame "Get Current Position" {
              n160 = Get Notifier Status(notifier=w551) -> (notifier out=w548:refnum<notifier>, current notification=w535:T8)  [unwired: 1 in, 3 out]
              n161 = Unbundle By Name(w535) -> ("CC Image (SGL)"=w523:T9, "CC Image Max (SGL)"=w518:T9)
              n162 = Unbundle By Name(w535) -> ("Ref FFT Stack (CSG)"=w526:T9[])
              n163 = Unbundle By Name(w535) -> ("No. of Frames"=w529:u32, "Cur Image (SGL)"=w537:T9, "Tmp Image FFT (CSG)"=w531:T9[])
              n164 = Unbundle By Name(w535) -> ("Sample Z (µm)"=w550:dbl[])
              n165 = To Unsigned Word Integer(number=w529) -> (unsigned 16bit integer=w528:u16)
              n166 = call "Generic Camera Get New Camera Image.vi"("Camera Notifier Name"=w538, "Frames"=w528) -> ("Image - U16"=w540:u16[][])  [unwired: 11 in, 2 out]
              n167 = Index Array(array=w531, index #1=0 ("index"), index #2=1 ("index"), index #3=2 ("index")) -> (element #1=w530:T9, element #2=w527:T9, element #3=w524:T9)
              n168 = To Single Precision Float(number=w540) -> (single precision float=w539:sgl[][])
              n169 = call "IMAQ ArrayToImage"("Image Pixels (Float)"=w539, "Image"=w537) -> ("Image Out"=w536:T9)  [unwired: 8 in, 1 out]
              n170 = call "4Pi Focus Lock - Norm FFT.vi"("FFT Image Dst"=w530, "Image In"=w536) -> ("FFT Image Out"=w546:T9)  [unwired: 8 in, 1 out]
              n171 = call "IMAQ ComplexConjugate"("Image Src"=w546) -> ("Image Dst Out"=w525:T9)  [unwired: 3 in, 1 out]
              n172 = for {
                tunnel: [w559] -> w521 mode=indexing
                shift-right: [w559] -> _
                shift-left: sgl 0.0 ("Max CC") -> [w560]
                tunnel: w523 -> [w553]
                tunnel: w527 -> [w557]
                tunnel: w526 -> [w556] mode=indexing
                tunnel: w525 -> [w555]
                tunnel: w524 -> [w554]
                tunnel: w518 -> [w552]
                n173 = call "4Pi Focus Lock - Get Cross Correlation.vi"("Ref FFT image"=w556, "Cur FFT Image"=w555, "FFT CC image"=w557, "iFFT image"=w554, "CC image"=w553) -> ("Max CC"=w559:sgl, "CC Image Out"=w558:T9)  [unwired: 8 in, 1 out]
                n174 = Greater?(x=w559, y=w560) -> (0:w561:bool)
                n175 = case shown="True" w561 {
                  tunnel: w552 -> [_ w563]
                  tunnel: w558 -> [_ w562]
                  frame False {
                  }
                  frame True {
                    n176 = call "IMAQ Copy"("Image Dst"=w563, "Image Src"=w562) -> ()  [unwired: 4 in, 2 out]
                  }
                }
              }
              n177 = To Double Precision Float(number=w521) -> (double precision float=w520:dbl[])
              n178 = call "4Pi Focus Lock - Find Peak Position.vi"("Fit Size"=2, "y"=w520, "x"=w550) -> ("Peak value"=→"cc max":dbl, "Coerced Peak Position"=w545:dbl)  [unwired: 6 in, 1 out]
              "Measured Z (µm)" <- w545
              n179 = Not A Number/Path/Refnum?(number/path/refnum=w545) -> (NaN/Path/Refnum?=w544:bool)
              n180 = Select(t=4Pi_Focus_Lock_-_Actions."Get Current Position", s=w544, f=4Pi_Focus_Lock_-_Actions."Get Current XY Position" ("y")) -> (s? t:f=w541:T7)
            }
            frame "Get Current XY Position" {
              w580 = 3 ("edge size")
              n181 = Get Notifier Status(notifier=w570) -> (notifier out=w566:refnum<notifier>, current notification=w569:T8)  [unwired: 1 in, 3 out]
              n182 = Unbundle By Name(w569) -> ("CC Image Max (SGL)"=w590:T9)
              n183 = call "IMAQ ImageToArray"("Image"=w590) -> ("Image Pixels (Float)"=w577:sgl[][])  [unwired: 3 in, 4 out]
              n184 = call "4Pi Focus Lock - FFT shift 2D.vi"("Input image"=w577) -> ("fft shifted image"=w576:sgl[][])  [unwired: 10 in]
              n185 = call "4Pi Focus Lock - Crop Imag at Max.vi"("edge size"=w580, "Input array"=w576) -> ("Y"=w586:i32, "X"=w587:i32, "subarray"=w589:sgl[][])  [unwired: 6 in, 1 out]
              n186 = To Double Precision Float(number=w589) -> (double precision float=w572:dbl[][])
              n187 = Build Array(w587, w586) -> (w585:i32[])
              n188 = call "4Pi Focus Lock - 2D Gaussian - Fit -init.vi"("Image In (DBL)"=w572, "width"=10.0) -> ("Best Fit Params"=w588:T17)  [unwired: 12 in, 1 out]
              n189 = To Double Precision Float(number=w585) -> (double precision float=w582:dbl[])
              n190 = Unbundle By Name(w588) -> ("X Position"=w584:dbl, "Y Position"=w583:dbl)
              n191 = Build Array(w584, w583) -> (w581:dbl[])
              n192 = To Double Precision Float(number=w580) -> (double precision float=w579:dbl)
              n193 = Subtract(x=w581, y=w579) -> (x-y=w578:dbl[])
              n194 = Add(x=w578, y=w582) -> (x+y=w573:dbl[])
              n195 = Index Array(array=w573, index #1=0 ("index"), index #2=1 ("index")) -> (element #1=→"Measured X Position cc (px)":dbl, element #2=→"Measured Y Position cc (px)":dbl)
            }
            frame "Get Current Position Gauss" {
              n196 = Get Notifier Status(notifier=w619) -> (notifier out=w618:refnum<notifier>, current notification=w616:T8)  [unwired: 1 in, 3 out]
              n197 = Unbundle By Name(w616) -> ("Cur Image (SGL)"=w615:T9)
              n198 = Unbundle By Name(w616) -> ("No. of Frames"=w613:u32)
              n199 = To Unsigned Word Integer(number=w613) -> (unsigned 16bit integer=w612:u16)
              n200 = call "Generic Camera Get New Camera Image.vi"("Camera Notifier Name"=w592, "Frames"=w612) -> ("Image - U16"=w599:u16[][])  [unwired: 11 in, 2 out]
              n201 = To Single Precision Float(number=w599) -> (single precision float=w617:sgl[][])
              n202 = call "IMAQ ArrayToImage"("Image Pixels (Float)"=w617, "Image"=w615) -> ()  [unwired: 8 in, 2 out]
              n203 = call "4Pi Focus Lock - 2D Gaussian - Fit Image U16.vi"("Image In (U16)"=w599) -> ("Best Fit Params"=w611:T17, "Error Out"=w607:errorcluster)  [unwired: 13 in]
              n204 = Unbundle By Name(w607) -> ("status"=w591:bool)
              n205 = Cluster To Array(cluster=w611) -> (array=w610:dbl[])
              n206 = Array Subset(array=w610, index=1, length=4) -> (w600:dbl[])
              n207 = Index Array(array=w600, index #1=0 ("index"), index #2=1 ("index"), index #3=2 ("index"), index #4=3 ("index")) -> (element #1=→"Measured X Position G (px)":dbl, element #2=→"Measured Y Position G (px)":dbl, element #3=w602:dbl, element #4=w601:dbl)
              n208 = Divide(x=w602, y=w601) -> (x/y=→"Measured sx/sy":dbl)
              n209 = Select(t=4Pi_Focus_Lock_-_Actions."Abort" ("y"), s=w591, f=4Pi_Focus_Lock_-_Actions."Check Drift" ("y")) -> (s? t:f=w593:T7)
            }
            frame "Get Current Position 1" {
              n210 = Get Notifier Status(notifier=w639) -> (notifier out=w634:refnum<notifier>, current notification=w638:T8)  [unwired: 1 in, 3 out]
              n211 = Unbundle By Name(w638) -> ("No. of Frames"=w621:u32, "Cur Image (SGL)"=w623:T9, "CC Image (SGL)"=w629:T9)
              n212 = Unbundle By Name(w638) -> ("Sample Z (µm)"=w637:dbl[])
              n213 = Unbundle By Name(w638) -> ("Ref Stack (SGL)"=w632:T9[])
              n214 = To Unsigned Word Integer(number=w621) -> (unsigned 16bit integer=w620:u16)
              n215 = call "Generic Camera Get New Camera Image.vi"("Camera Notifier Name"=w624, "Frames"=w620) -> ("Image - U16"=w626:u16[][])  [unwired: 11 in, 2 out]
              n216 = To Single Precision Float(number=w626) -> (single precision float=w625:sgl[][])
              n217 = call "IMAQ ArrayToImage"("Image Pixels (Float)"=w625, "Image"=w623) -> ("Image Out"=w622:T9)  [unwired: 8 in, 1 out]
              n218 = call "4Pi Focus Lock - Img Norm.vi"("Image In"=w622) -> ("Image Dst Out"=w630:T9)  [unwired: 9 in, 1 out]
              n219 = for {
                tunnel: w632 -> [w650] mode=indexing
                tunnel: w630 -> [w648]
                tunnel: w629 -> [w647]
                tunnel: [w646] -> w628 mode=indexing
                n220 = call "4Pi Focus Lock - Img Norm.vi"("Image In"=w650) -> ("Image Dst Out"=w649:T9)  [unwired: 9 in, 1 out]
                n221 = call "IMAQ Multiply"("Image Src A"=w649, "Image Dst"=w647, "Image Src B"=w648) -> ("Image Dst Out"=w645:T9)  [unwired: 4 in, 1 out]
                n222 = call "IMAQ ImageToArray"("Image"=w645) -> ("Image Pixels (Float)"=w644:sgl[][])  [unwired: 3 in, 4 out]
                n223 = Add Array Elements(numeric array=w644) -> (sum=w642:sgl)
                n224 = Array Size(array=w644) -> (size(s)=w643:i32[])
                n225 = Multiply Array Elements(1:w643) -> (0:w641:i32)
                n226 = To Double Precision Float(number=w641) -> (double precision float=w640:dbl)
                n227 = Divide(x=w642, y=w640) -> (x/y=w646:dbl)
              }
              n228 = To Double Precision Float(number=w628) -> (double precision float=w631:dbl[])
              n229 = call "4Pi Focus Lock - Find Peak Position.vi"("Fit Size"=2, "y"=w631, "x"=w637) -> ("Coerced Peak Position"=w627:dbl)  [unwired: 6 in, 2 out]
              n230 = local write "Measured Z (µm)"(w627) -> ()
            }
            frame "Check Drift" {
              n231 = Get Notifier Status(notifier=w668) -> (notifier out=w661:refnum<notifier>, current notification=w667:T8)  [unwired: 1 in, 3 out]
              n232 = Unbundle By Name(w667) -> ("Z Correction Active"=w654:bool, "Z Drift Threshold"=w662:dbl, "PID Values"=w666:dbl[])
              n233 = local read "Measured Z (µm)"() -> (w657:dbl)
              n234 = local read "Target Z (µm)"() -> (w658:dbl)
              n235 = Array To Cluster(array=w666) -> (cluster=w665:T18)
              n236 = Subtract(x=w658, y=w657) -> (x-y=w659:dbl)
              n237 = call-poly <vilib>:"PID.vi"("PID gains"=w665, "process variable"=w657, "setpoint"=w658) -> ("dt out (s)"=→"dt (s)":dbl, "output"=→"dz":dbl)  [unwired: 7 in]
              n238 = Absolute Value(x=w659) -> (abs(x)=w656:dbl)
              n239 = Greater?(x=w656, y=w662) -> (0:w655:bool)
              n240 = And(x=w654, y=w655) -> (x .and. y?=w653:bool)
              n241 = case shown="False" w653 {
                tunnel: [4Pi_Focus_Lock_-_Actions."Update Plots" ("y") 4Pi_Focus_Lock_-_Actions."Move Z" ("y")] -> w651
                tunnel: [FALSE TRUE] -> w652
                frame False {
                }
                frame True {
                }
              }
              "Z Move" <- w652
            }
            frame "Check Drift Gauss" {
              n242 = Get Notifier Status(notifier=w692) -> (notifier out=w688:refnum<notifier>, current notification=w691:T8)  [unwired: 1 in, 3 out]
              n243 = Unbundle By Name(w691) -> ("Z Correction Active"=w681:bool, "Z Drift Threshold"=w676:dbl, "PID Values"=w690:dbl[])
              n244 = local read "Measured sx/sy"() -> (w684:dbl)
              n245 = local read "Target sx/sy"() -> (w685:dbl)
              n246 = Array To Cluster(array=w690) -> (cluster=w689:T18)
              n247 = Subtract(x=w685, y=w684) -> (x-y=w686:dbl)
              n248 = call-poly <vilib>:"PID.vi"("PID gains"=w689, "process variable"=w684, "setpoint"=w685) -> ("dt out (s)"=w678:dbl, "output"=w679:dbl)  [unwired: 7 in]
              n249 = Divide(x=w676, y="Metric scale sx/sy") -> (x/y=w674:dbl)
              n250 = Absolute Value(x=w686) -> (abs(x)=w683:dbl)
              n251 = local write "dz"(w679) -> ()
              n252 = local write "dt (s)"(w678) -> ()
              n253 = Greater?(x=w683, y=w674) -> (0:w682:bool)
              n254 = And(x=w681, y=w682) -> (x .and. y?=w677:bool)
              n255 = case shown="False" w677 {
                tunnel: [4Pi_Focus_Lock_-_Actions."Update Plots" ("y") 4Pi_Focus_Lock_-_Actions."Move Z" ("y")] -> w680
                tunnel: [FALSE TRUE] -> w673
                frame False {
                }
                frame True {
                }
              }
              n256 = local write "Z Move"(w673) -> ()
            }
            frame "Move Z" {
              n257 = Get Notifier Status(notifier=w712) -> (notifier out=w705:refnum<notifier>, current notification=w711:T8)  [unwired: 1 in, 3 out]
              n258 = Unbundle By Name(w711) -> ("Z Stage Move Limit (µm)"=w709:dbl)
              n259 = local read "dz"() -> (w710:dbl)
              n260 = Multiply(x=w710, y="Update Scale Factor") -> (x*y=w703:dbl)
              n261 = Absolute Value(x=w703) -> (abs(x)=w708:dbl)
              n262 = Greater?(x=w709, y=w708) -> (0:w699:bool)
              n263 = local read "Z Move"() -> (w701:bool)
              n264 = And(x=w699, y=w701) -> (x .and. y?=w702:bool)
              n265 = case shown="True" w702 {
                tunnel: w703 -> [_ w714]
                tunnel: w707 -> [_ w713]
                frame False {
                }
                frame True {
                  n266 = Build Array(w714) -> (w715:dbl[])
                  n267 = flat-sequence {
                    tunnel: w715 -> [w719]
                    tunnel: w713 -> [w717]
                    frame #0 {
                      n268 = call "Stages Messenger.vi"("Stage Notifier Name"=w717, "Actions"=Stage_Actions."MVR", "Setpoint"=w719, "Axis"=bool[] [TRUE], "Exit While Busy?"=FALSE) -> ()  [unwired: 6 in, 5 out]
                    }
                    frame #1 {
                      n269 = Wait (ms)(milliseconds to wait=u32 350) -> ()  [unwired: 1 out]
                    }
                  }
                }
              }
              n270 = Select(t=4Pi_Focus_Lock_-_Actions."Update Plots" ("y"), s=w699, f=4Pi_Focus_Lock_-_Actions."Abort") -> (s? t:f=w697:T7)
            }
            frame "Update Plots" {
              n271 = Get Notifier Status(notifier=w771) -> (notifier out=w760:refnum<notifier>, current notification=w769:T8)  [unwired: 1 in, 3 out]
              n272 = local read "Measured sx/sy"() -> (w742:dbl)
              n273 = local read "Target sx/sy"() -> (w741:dbl)
              n274 = Unbundle By Name(w769) -> ("Z Drift Threshold"=w770:dbl)
              n275 = Unbundle By Name(w769) -> ("Initial Z Position (µm)"=w768:dbl)
              n276 = local read "Measured Z (µm)"() -> (w740:dbl)
              n277 = local read "Metric scale sx/sy"() -> (w738:dbl)
              n278 = local read "Target Z (µm)"() -> (w772:dbl)
              n279 = Subtract(x=w742, y=w741) -> (x-y=w739:dbl)
              n280 = call "Stages Messenger.vi"("Stage Notifier Name"=w737, "Actions"=Stage_Actions."Get Position", "Exit While Busy?"=TRUE) -> ("Positions"=w762:dbl[])  [unwired: 8 in, 4 out]
              n281 = Multiply(x=w739, y=w738) -> (x*y=w736:dbl)
              n282 = Index Array(array=w762, index=0) -> (element=w761:dbl)
              n283 = Subtract(x=w761, y=w768) -> (x-y=w767:dbl)
              n284 = local write "Stage Position (µm)"(w761) -> ()
              n285 = call "4Pi Focus Lock - Values Organize Plot Data.vi"("Target 01"=w772, "Value Limit"=w770, "Current 1"=w740, "Current 2"=w736, "Stage Position"=w767) -> ("output cluster"=→"Z Target and Fit Value (µm)":T1)  [unwired: 10 in]
              n286 = local read "Measured X Position cc (px)"() -> (w752:dbl)
              n287 = local read "Measured Y Position cc (px)"() -> (w751:dbl)
              n288 = local read "Target X Position cc (px)"() -> (w750:dbl)
              n289 = local read "Target Y Position cc (px)"() -> (w749:dbl)
              n290 = local read "Measured Y Position G (px)"() -> (w731:dbl)
              n291 = local read "Measured X Position G (px)"() -> (w732:dbl)
              n292 = local read "Target X Position G (px)"() -> (w730:dbl)
              n293 = local read "Target Y Position G (px)"() -> (w729:dbl)
              n294 = Build Array(w732, w731) -> (w734:dbl[])
              n295 = Build Array(w730, w729) -> (w735:dbl[])
              n296 = Build Array(w752, w751) -> (w756:dbl[])
              n297 = Build Array(w750, w749) -> (w757:dbl[])
              n298 = Subtract(x=w734, y=w735) -> (x-y=w733:dbl[])
              n299 = Subtract(x=w756, y=w757) -> (x-y=w748:dbl[])
              n300 = Multiply(x=w733, y="Pixe Size in XY (µm)") -> (x*y=w725:dbl[])
              n301 = Multiply(x=w748, y="Pixe Size in XY (µm)") -> (x*y=w755:dbl[])
              n302 = local read "cc max"() -> (w744:dbl)
              n303 = Index Array(array=w725, index #1=0 ("index"), index #2=1 ("index")) -> (element #1=w724:dbl, element #2=w723:dbl)
              n304 = Index Array(array=w755, index #1=0 ("index"), index #2=1 ("index")) -> (element #1=w747:dbl, element #2=w746:dbl)
              n305 = Bundle("cc max"=w744) -> (→"CC Max":cluster{" cc max":dbl})  [unwired: 1 in]
              n306 = Bundle(w724, w723, w747, w746, 0.0) -> (→"X Y Fit Value (µm)":cluster{dbl, dbl, dbl, dbl, dbl})  [unwired: 1 in]
            }
            frame "Abort" {
              n307 = Get Notifier Status(notifier=w778) -> (notifier out=w783:refnum<notifier>, current notification=w782:T8)  [unwired: 1 in, 3 out]
              n308 = call "Camera Messenger.vi"("Notifier Name"=w777, "General Camera Actions"=Generic_Camera_Actions."Abort") -> ()  [unwired: 8 in, 6 out]
              n309 = Bundle By Name(cluster=w782, "Running?"=FALSE, "Actions"=4Pi_Focus_Lock_-_Actions."Exit Loop") -> (w780:T8)
              n310 = Send Notification(notification=w780, notifier=w783) -> (notifier out=w774:refnum<notifier>)  [unwired: 1 in, 1 out]
            }
            frame "Exit Loop" {
            }
            frame "Quit" {
              n311 = Get Notifier Status(notifier=w788) -> (current notification=w794:T8)  [unwired: 1 in, 4 out]
              n312 = Unbundle By Name(w794) -> ("Ref Stack (SGL)"=w793:T9[], "Cur Image (SGL)"=w792:T9, "Tmp Image FFT (CSG)"=w791:T9[], "CC Image (SGL)"=w790:T9, "Ref FFT Stack (CSG)"=w787:T9[])
              n313 = Build Array (concatenate)(w793, w792, w791, w790, w787) -> (w789:T9[])
              n314 = for {
                tunnel: w789 -> [w797] mode=indexing
                n315 = call "IMAQ Dispose"("Image"=w797) -> ()  [unwired: 5 in, 1 out]
              }
            }
          }
          n316 = Get Notifier Status(notifier=w301) -> (current notification=w309:T8)  [unwired: 1 in, 4 out]
          n317 = Unbundle By Name(w309) -> ("Actions"=w308:T7)
          n318 = Equal?(x=w306, y=w308) -> (x = y?=w307:bool)
          n319 = Select(t=w306, s=w307, f=w305) -> (s? t:f=w304:T7)
        }
      }
      n320 = while {
        tunnel: w149 -> [w164]
        tunnel: w153 -> [w163]
        stop <- w162 stop-if-true
        n321 = event shown="[1] \"Set Camera ROI\", \"Camera Settings\": Value Change" {
          selector: _ -> [_ _ _ _ _ _ _]
          dyn-events: _ -> [_ _ _ _ _ _ _]
          timeout: -1 -> [_ _ _ _ _ _ _]
          tunnel: w164 -> [_ w166 _ _ _ _ _]
          tunnel: w163 -> [_ _ w185 w223 w251 w262 w266]
          tunnel: [w165 w169 w176 w220 w245 w256 w264] -> w162
          tunnel: FALSE ("NewVal") -> [w165 w169 w176 w220 w245 w256 _]
          event Timeout {
            n322 = event-data() -> ()  [unwired: 1 in, 3 out]
          }
          event "Set Camera ROI", "Camera Settings": Value Change {
            n323 = event-data() -> ("CtlRef"=w168:refnum<vi>)  [unwired: 1 in]
            n324 = property class="Bool"(reference=w168) -> ("Label.Text"=w167:string)  [unwired: 1 in, 2 out]
            n325 = case shown="\"Camera Settings\"" w167 {
              tunnel: w166 -> [_ w170 w175]
              frame Default {
              }
              frame "Camera Settings" {
                n326 = Select(t=Common_Device_Actions."Open Front Panel" ("Common Action"), s="Camera Settings", f=Common_Device_Actions."Close Front Panel") -> (s? t:f=w171:T13)
                n327 = call "Common Device Queue Messenger.vi"("Common Action"=w171, "Notifier Name"=w170) -> ()  [unwired: 13 in, 1 out]
              }
              frame "Set Camera ROI" {
                n328 = call "4Pi Focus Lock - Setup Camera.vi"("Camera Notifier Name"=w175) -> ()  [unwired: 14 in, 1 out]
              }
            }
          }
          event "P (Proportional)", "I (Integral)", "D (Derivative)", "Sample Z Step Size (µm)", "Z Move Limit (µm)", "Z Drift Threshold (µm)": Value Change {
            n329 = event-data() -> ("NewVal"=w180:dbl, "CtlRef"=w182:refnum<vi>)  [unwired: 1 in]
            n330 = Get Notifier Status(notifier=w185) -> (notifier out=w184:refnum<notifier>, current notification=w183:T8)  [unwired: 1 in, 3 out]
            n331 = property class="DigNum (strict)"(reference=w182) -> ("Label.Text"=w181:string)  [unwired: 1 in, 2 out]
            n332 = case shown="Default" w181 {
              tunnel: w183 -> [w186 w189 w195 w201 w207 w210 w213]
              tunnel: w180 -> [_ w190 w196 w202 w206 w209 w212]
              tunnel: [w186 w187 w193 w199 w205 w208 w211] -> w179
              frame Default {
              }
              frame "P (Proportional)" {
                n333 = Unbundle By Name(w189) -> ("PID Values"=w191:dbl[])
                n334 = Replace Array Subset(array=w191, new element=w190, index=0) -> (w188:dbl[])
                n335 = Bundle By Name(cluster=w189, "PID Values"=w188) -> (w187:T8)
              }
              frame "I (Integral)" {
                n336 = Unbundle By Name(w195) -> ("PID Values"=w197:dbl[])
                n337 = Replace Array Subset(array=w197, new element=w196, index=1) -> (w194:dbl[])
                n338 = Bundle By Name(cluster=w195, "PID Values"=w194) -> (w193:T8)
              }
              frame "D (Derivative)" {
                n339 = Unbundle By Name(w201) -> ("PID Values"=w203:dbl[])
                n340 = Replace Array Subset(array=w203, new element=w202, index=2) -> (w200:dbl[])
                n341 = Bundle By Name(cluster=w201, "PID Values"=w200) -> (w199:T8)
              }
              frame "Sample Z Step Size (µm)" {
                n342 = Bundle By Name(cluster=w207, "Z Step Size (µm)"=w206) -> (w205:T8)
              }
              frame "Z Move Limit (µm)" {
                n343 = Bundle By Name(cluster=w210, "Z Stage Move Limit (µm)"=w209) -> (w208:T8)
              }
              frame "Z Drift Threshold (µm)" {
                n344 = Bundle By Name(cluster=w213, "Z Drift Threshold"=w212) -> (w211:T8)
              }
            }
            n345 = Bundle By Name(cluster=w179, "Actions"=4Pi_Focus_Lock_-_Actions."Idle") -> (w177:T8)
            n346 = Send Notification(notification=w177, notifier=w184) -> ()  [unwired: 1 in, 2 out]
          }
          event "Sample Z Step No.", "Frame Accumulation": Value Change {
            n347 = event-data() -> ("NewVal"=w219:u32, "CtlRef"=w215:refnum<vi>)  [unwired: 1 in]
            n348 = property class="DigNum (strict)"(reference=w215) -> ("Label.Text"=w214:string)  [unwired: 1 in, 2 out]
            n349 = Get Notifier Status(notifier=w223) -> (notifier out=w221:refnum<notifier>, current notification=w222:T8)  [unwired: 1 in, 3 out]
            n350 = case shown="\"Frame Accumulation\"" w214 {
              tunnel: w222 -> [w224 w229 w244]
              tunnel: [w224 w228 w242] -> w218
              tunnel: w219 -> [_ w227 w243]
              frame Default {
              }
              frame "Sample Z Step No." {
                n351 = for {
                  N: w227 -> [_]
                  tunnel: [w241] -> w226 mode=indexing
                  tunnel: [w230] -> w225 mode=indexing
                  i -> [w240]
                  w231 = T10 3 items=["Grayscale (U8)", "Grayscale (I16)", "Grayscale (SGL)", "Complex (CSG)", "RGB (U32)", "HSL (U32)", "RGB (U64)", "Grayscale (U16)"] ("Image Type")
                  w236 = T10 2 items=["Grayscale (U8)", "Grayscale (I16)", "Grayscale (SGL)", "Complex (CSG)", "RGB (U32)", "HSL (U32)", "RGB (U64)", "Grayscale (U16)"] ("Image Type")
                  w232 = 10 ("Border Size")
                  n352 = Number To Decimal String(number=w240, width (-)=i16 1) -> (decimal integer string=w238:string)
                  n353 = Concatenate Strings("Ref Stack " ("string"), w238) -> (w234:string)
                  n354 = call "IMAQ Create"("Border Size"=w232, "Image Name"=w234, "Image Type"=w236) -> ("New Image"=w241:T9)  [unwired: 2 in, 1 out]
                  n355 = Concatenate Strings("FFT" ("string"), w234) -> (w233:string)
                  n356 = call "IMAQ Create"("Border Size"=w232, "Image Name"=w233, "Image Type"=w231) -> ("New Image"=w230:T9)  [unwired: 2 in, 1 out]
                }
                n357 = Bundle By Name(cluster=w229, "Z Step No."=w227, "Ref Stack (SGL)"=w226, "Ref FFT Stack (CSG)"=w225) -> (w228:T8)
              }
              frame "Frame Accumulation" {
                n358 = Bundle By Name(cluster=w244, "No. of Frames"=w243) -> (w242:T8)
              }
            }
            n359 = Bundle By Name(cluster=w218, "Actions"=4Pi_Focus_Lock_-_Actions."Idle") -> (w216:T8)
            n360 = Send Notification(notification=w216, notifier=w221) -> ()  [unwired: 1 in, 2 out]
          }
          event "Z Correction Active": Value Change {
            n361 = event-data() -> ("NewVal"=w249:bool)  [unwired: 1 in, 1 out]
            n362 = Get Notifier Status(notifier=w251) -> (notifier out=w247:refnum<notifier>, current notification=w250:T8)  [unwired: 1 in, 3 out]
            n363 = Bundle By Name(cluster=w250, "Actions"=4Pi_Focus_Lock_-_Actions."Idle", "Z Correction Active"=w249) -> (w246:T8)
            n364 = Send Notification(notification=w246, notifier=w247) -> ()  [unwired: 1 in, 2 out]
          }
          event "Start Lock": Value Change {
            n365 = event-data() -> ("NewVal"=w254:bool)  [unwired: 1 in]
            n366 = Select(t=4Pi_Focus_Lock_-_Actions."Start Lock", s=w254, f=4Pi_Focus_Lock_-_Actions."Abort" ("t")) -> (s? t:f=w259:T7)
            n367 = Select(t=TRUE ("Running?"), s=w254, f=FALSE) -> (s? t:f=w252:bool)
            n368 = Get Notifier Status(notifier=w262) -> (notifier out=w263:refnum<notifier>, current notification=w261:T8)  [unwired: 1 in, 3 out]
            n369 = Bundle By Name(cluster=w261, "Actions"=w259, "Running?"=w252) -> (w260:T8)
            n370 = Send Notification(notification=w260, notifier=w263) -> ()  [unwired: 1 in, 2 out]
          }
          event "Quit": Value Change {
            # "Turn off the Focus lock before quiting."
            n371 = event-data() -> ("NewVal"=w264:bool)  [unwired: 1 in]
            n372 = Get Notifier Status(notifier=w266) -> (notifier out=w269:refnum<notifier>, current notification=w267:T8)  [unwired: 1 in, 3 out]
            n373 = Unbundle By Name(w267) -> ("Running?"=w270:bool)
            n374 = case shown="False" w270 {
              tunnel: w269 -> [w274 w279]
              tunnel: [w274 w276] -> w268
              tunnel: w267 -> [_ w280]
              frame False {
              }
              frame True {
                n375 = Bundle By Name(cluster=w280, "Actions"=4Pi_Focus_Lock_-_Actions."Abort") -> (w278:T8)
                n376 = Send Notification(notification=w278, notifier=w279) -> (notifier out=w277:refnum<notifier>)  [unwired: 1 in, 1 out]
                n377 = while {
                  tunnel: w277 -> [w290]
                  tunnel: [w285] -> w276
                  i -> [w284]
                  stop <- w286 stop-if-true
                  n378 = Get Notifier Status(notifier=w290) -> (notifier out=w285:refnum<notifier>, # waiting=w289:i32)  [unwired: 1 in, 3 out]
                  n379 = Greater?(x=w284, y=1500) -> (0:w282:bool)
                  n380 = Less?(x=w289, y=1) -> (x < y?=w287:bool)
                  n381 = Or(x=w287, y=w282) -> (x .or. y?=w286:bool)
                  n382 = Wait (ms)(milliseconds to wait=u32 1) -> ()  [unwired: 1 out]
                }
              }
            }
            n383 = Get Notifier Status(notifier=w268) -> (notifier out=w272:refnum<notifier>, current notification=w273:T8)  [unwired: 1 in, 3 out]
            n384 = Bundle By Name(cluster=w273, "Actions"=4Pi_Focus_Lock_-_Actions."Quit") -> (w271:T8)
            n385 = Send Notification(notification=w271, notifier=w272) -> ()  [unwired: 1 in, 2 out]
          }
        }
      }
      n386 = Release Notifier(notifier=w151, force destroy? (F)=TRUE) -> ()  [unwired: 1 in, 3 out]
    }
    frame Error {
    }
  }
  n387 = control-ref of="This VI"() -> (w32:refnum<vi>)
  n388 = property class="VI"(reference=w32) -> (reference out=w40:refnum<vi>, "Panel"=w33:refnum<vi>)  [unwired: 1 in, 1 out]
  n389 = property class="Pnl"(reference=w33) -> ("Decos[]"=w31:refnum<vi>[], "Panes[]"=w36:refnum<vi>[])  [unwired: 1 in, 2 out]
  n390 = Array Size(array=w31) -> (size(s)=w29:i32)
  n391 = Decrement(x=w29) -> (x-1=w30:i32)
  n392 = Index Array(array=w36, index=0) -> (element=w35:refnum<vi>)
  n393 = Index Array(array=w31, index=w30) -> (element=w38:refnum<vi>)
  n394 = property class="VI"(reference=w40) -> (reference out=w42:refnum<vi>, "Front Panel.PanelBounds"=w43:T19)  [unwired: 1 in, 1 out]
  n395 = property class="Decor"(reference=w38) -> ("Bounds"=w41:T20)  [unwired: 1 in, 2 out]
  n396 = property class="Pane"(reference=w35, "Origin"=T6 {"Horizontal"=0, "Vertical"=0}, "HorizScrollbarVisibility"=w39, "VertScrollbarVisibility"=w39) -> ()  [unwired: 1 in, 2 out]
  n397 = control-ref of="Quit"() -> (w28:refnum<vi>)
  n398 = Unbundle By Name(w41) -> ("Width"=w46:u32, "Height"=w49:u32)
  n399 = To Word Integer(number=w46) -> (16bit integer=w48:i16)
  n400 = To Word Integer(number=w49) -> ()  [unwired: 1 out]
  n401 = property class="Bool"(reference=w28) -> ("Height"=w51:u32, "Top"=w52:i32)  [unwired: 1 in, 2 out]
  n402 = Unbundle By Name(w43) -> ("Left"=w45:i16, "Top"=w56:i16)
  n403 = To Word Integer(number=w51) -> (16bit integer=w54:i16)
  n404 = To Word Integer(number=w52) -> (16bit integer=w55:i16)
  n405 = Add(x=w45, y=w48) -> (x+y=w47:i16)
  n406 = Compound Arithmetic op=ADD(w56, w54, w55, i16 12 ("y")) -> (w50:i16)
  n407 = Bundle By Name(cluster=w43, "Right"=w47, "Bottom"=w50) -> (w44:T19)
  n408 = property class="VI"(reference=w42, "Front Panel.PanelBounds"=w44) -> ()  [unwired: 1 in, 2 out]
